vi "Create Mesh with Attributes.vi"(0 "Draw Mode":T4(ring), 1 "Color Binding Mode":T3(ring), 2 "Color Array":T2(array[cluster]), 5 "Vertex Array":cluster{"X":sgl, "Y":sgl, "Z":sgl}[](array[cluster]), 7 "Indices":u32[](array[numeric]), 9 "Normal Array":cluster{"X":sgl, "Y":sgl, "Z":sgl}[](array[cluster]), 11 "error in (no error)":errorcluster, 12 "Normal Binding Mode":T3(ring), 13 "Texture Coordinate Array":T1) -> (4 "New Mesh Refnum":refnum<vi>, 15 "error out":errorcluster)   [LabVIEW 2017, in "NI_3D Picture Control.lvlib"]
doc: "Creates a mesh with customizable color and draw options."
uses:
  <vilib>/picture/3D Picture Control/NI_3D Picture Control.lvlib
  <vilib>/Utility/miscctls.llb/LVTextureCoordinateArrayTypeDef.ctl
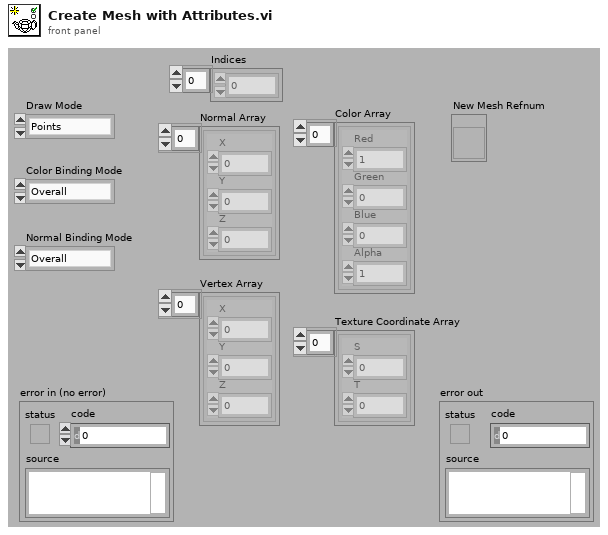
[diagram p1: front panel]
types:
  T1 = typedef "LVTextureCoordinateArrayTypeDef.ctl" = cluster{"S":sgl, "T":sgl}[]
  T2 = cluster{"Red":sgl, "Green":sgl, "Blue":sgl, "Alpha":sgl}[]
  T3 = enum16{"Overall", "Per Primitive", "Per Vertex", "Binding Off"}
  T4 = enum16{"Points", "Lines", "Line Strip", "Line Loop", "Triangles", "Triangle Strip", "Triangle Fan", "Quads", "Quad Strip", "Polygon"}
  T5 = cluster{"Red":sgl, "Green":sgl, "Blue":sgl, "Alpha":sgl}
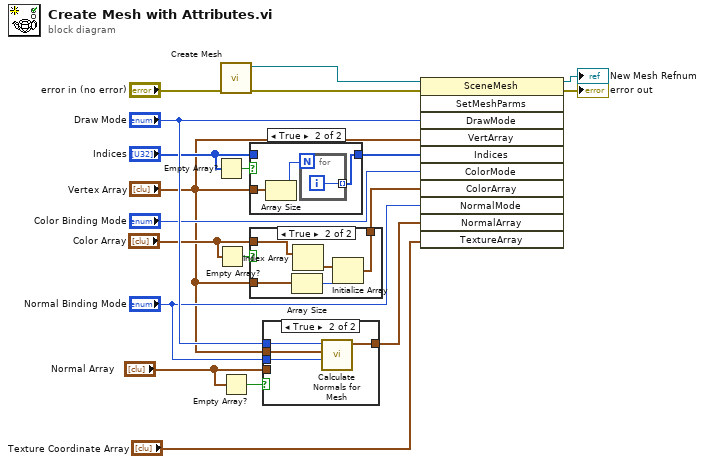
[diagram p0: block diagram]
diagram:
  n1 = Empty Array?(array="Indices") -> (empty?=w9:bool)
  n2 = Empty Array?(array="Color Array") -> (empty?=w2:bool)
  n3 = call <vilib>:"Create Mesh.vi"("error in (no error)"="error in (no error)") -> ("error out"=w17:errorcluster, "New Mesh Refnum"=w19:refnum<vi>)  [unwired: 9 out]
  n4 = Empty Array?(array="Normal Array") -> (empty?=w13:bool)
  n5 = case shown="True" w9 {
    tunnel: "Indices" -> [w20 _]
    tunnel: [w20 w21] -> w1
    tunnel: "Vertex Array" -> [_ w23]
    frame False {
    }
    frame True {
      n6 = Array Size(array=w23) -> (size(s)=w22:i32)
      n7 = for {
        N: w22 -> [_]
        tunnel: [w24] -> w21 mode=indexing
        i -> [w24]
      }
    }
  }
  n8 = case shown="True" w2 {
    tunnel: "Color Array" -> [w25 w29]
    tunnel: [w25 w27] -> w5
    tunnel: "Vertex Array" -> [_ w26]
    frame False {
    }
    frame True {
      n9 = Array Size(array=w26) -> (size(s)=w30:i32)
      n10 = Index Array(array=w29) -> (element=w28:T5)  [unwired: 1 in]
      n11 = Initialize Array(w28, w30) -> (w27:T2)
    }
  }
  n12 = case shown="True" w13 {
    tunnel: "Draw Mode" -> [_ w35]
    tunnel: "Vertex Array" -> [_ w34]
    tunnel: "Normal Binding Mode" -> [_ w33]
    tunnel: [w31 w32] -> w12
    tunnel: "Normal Array" -> [w31 _]
    frame False {
    }
    frame True {
      n13 = call <vilib>:"Calculate Normals for Mesh.vi"("Color Binding Mode"=w33, "Vertex Array"=w34, "Draw Mode"=w35) -> ("Normal Array"=w32:cluster{"X":sgl, "Y":sgl, "Z":sgl}[])  [unwired: 8 in]
    }
  }
  n14 = invoke class="SceneMesh" method="SetMeshParms"(reference=w19, error in=w17, "DrawMode"="Draw Mode", "VertArray"="Vertex Array", "Indices"=w1, "ColorMode"="Color Binding Mode", "ColorArray"=w5, "NormalMode"="Normal Binding Mode", "NormalArray"=w12, "TextureArray"="Texture Coordinate Array") -> (reference out=→"New Mesh Refnum":refnum<vi>, error out=→"error out":errorcluster)  [unwired: 1 in, 9 out]
